vi "dfd_nMAC_CoefMap.vi"(9 "chCnt":u16, 10 "coefSetIdx":u16, 11 "coefOffsetAddr":u16) -> (3 "coefRDAddr":u16)   [LabVIEW 2017]
uses:
  <vilib>/rvi/FXPMathLib/basic elements/FxpDiscreteDelay/XNode/nifxpmath_DiscreteDelay.xnode
  <vilib>/rvi/FXPMathLib/basic elements/FxpAddSub/XNode/nifxpmath_AddSub.xnode
  <vilib>/rvi/FXPMathLib/sim/FxpSim.dll
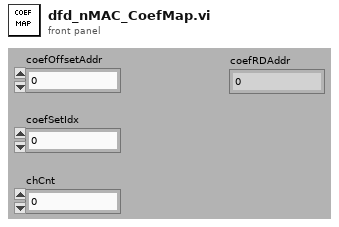
[diagram p1: front panel]
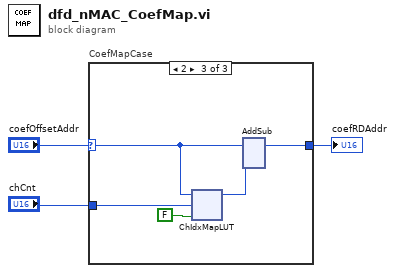
[diagram p0: block diagram]
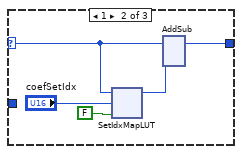
[diagram p3: hidden frame]
diagram:
  n1 = case "CoefMapCase" shown="2" "coefOffsetAddr" {
    selector: "coefOffsetAddr" -> [w4 w8 w62]
    tunnel: [w4 w6 w60] -> w2
    tunnel: "chCnt" -> [_ _ w59]
    frame 0, Default {
    }
    frame 1 {
      n2 = xnode "SetIdxMapLUT"("D"=w8, "n-1[0..15]"="coefSetIdx", "enable"=FALSE) -> ("Q"=w7:u16)
      n3 = xnode "AddSub"("x"=w8, "y"=w7) -> ("s"=w6:u16)  [unwired: 1 out]
    }
    frame 2 {
      n4 = xnode "ChIdxMapLUT"("D"=w62, "n-1[0..15]"=w59, "enable"=FALSE) -> ("Q"=w61:u16)
      n5 = xnode "AddSub"("x"=w62, "y"=w61) -> ("s"=w60:u16)  [unwired: 1 out]
    }
  }
  "coefRDAddr" <- w2
